vi "IMG_FW_UIS_SetPanelOrigin.vi"(8 "error in (no error)":errorcluster, 9 "minimum size":cluster{"Width":i16, "Height":i16}, 10 "origin":T1, 11 "reference":refnum<vi>) -> (0 "error out":errorcluster)   [LabVIEW 2016]
uses:
  <vilib>/Utility/miscctls.llb/LVPointTypeDef.ctl
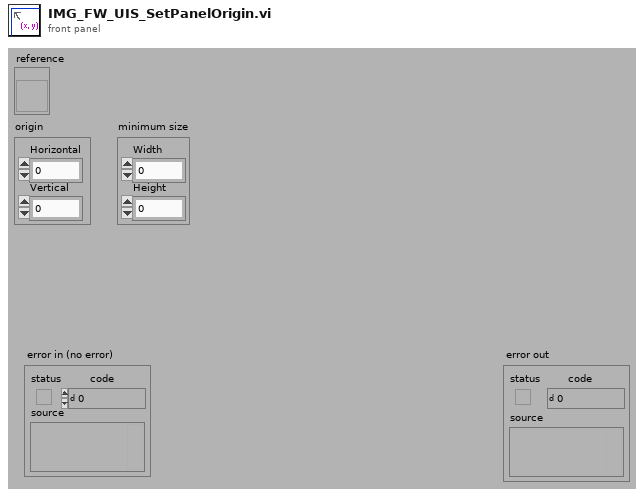
[diagram p1: front panel]
types:
  T1 = typedef "LVPointTypeDef.ctl" = cluster{"Horizontal":i16, "Vertical":i16}
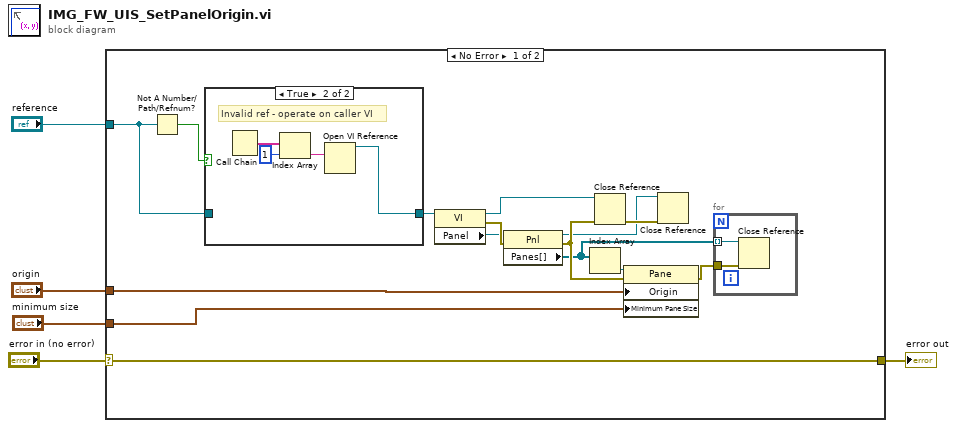
[diagram p0: block diagram]
diagram:
  n1 = case shown="No Error" "error in (no error)" {
    selector: "error in (no error)" -> [w20 w28]
    tunnel: [w20 w28] -> w4
    tunnel: "origin" -> [w8 _]
    tunnel: "reference" -> [w12 _]
    tunnel: "minimum size" -> [w6 _]
    frame No Error {
      n2 = Not A Number/Path/Refnum?(number/path/refnum=w12) -> (NaN/Path/Refnum?=w13:bool)
      n3 = case shown="True" w13 {
        tunnel: [w21 w22] -> w11
        tunnel: w12 -> [w21 _]
        frame False {
        }
        frame True {
          # "Invalid ref - operate on caller VI"
          n4 = Call Chain() -> (call chain=w25:string[])
          n5 = Index Array(array=w25, index=1) -> (element=w23:string)
          n6 = Open VI Reference(vi path=w23) -> (vi reference=w22:refnum<vi>)  [unwired: 1 in, 5 out]
        }
      }
      n7 = property on="Property Node" class="VI"(reference=w11) -> (reference out=w15:refnum<vi>, error out=w18:errorcluster, "Panel"=w7:refnum<vi>)  [unwired: 1 in]
      n8 = property on="Property Node" class="Pnl"(reference=w7, error in=w18) -> (reference out=w9:refnum<vi>, error out=w16:errorcluster, "Panes[]"=w14:refnum<vi>[])
      n9 = Index Array(array=w14) -> (element=w19:refnum<vi>)  [unwired: 1 in]
      n10 = Close Reference(reference=w15, error in (no error)=w16) -> (error out=w10:errorcluster)
      n11 = property on="Property Node" class="Pane"(reference=w19, error in=w16, "Origin"=w8, "Minimum Pane Size"=w6) -> (error out=w17:errorcluster)  [unwired: 1 out]
      n12 = Close Reference(reference=w9, error in (no error)=w10) -> ()  [unwired: 1 out]
      n13 = for {
        tunnel: w14 -> [w27] mode=indexing
        tunnel: w17 -> [w26]
        n14 = Close Reference(reference=w27, error in (no error)=w26) -> ()  [unwired: 1 out]
      }
    }
    frame Error {
    }
  }
  "error out" <- w4
